vi "ExTestAdvDisp.vi"() -> ()   [LabVIEW 2010]
panel:
  out "After Pin zoom y":dbl format="%.2f"
  out "After Pin zoom x":dbl format="%.2f"
  out "zoom y":dbl format="%.2f"
  out "Zoom x":dbl format="%.2f"
  out "Cursor Y":u32
  out "Cursor X":u32
  in  "Full File Name":path
  out "error out":errorcluster
  in  "error in (no error)":errorcluster
  in  "SITKFULLDISPLAYLib.SITKFullDisplay":refnum<k7>(container)
  # "Browse match pattern is set to *.tif.  Modify this if different file type is needed."
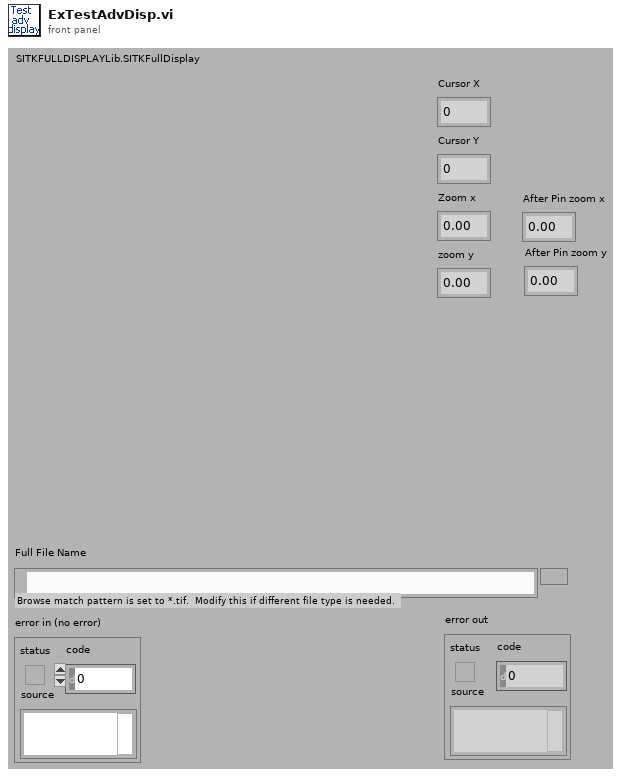
[diagram p1: front panel]
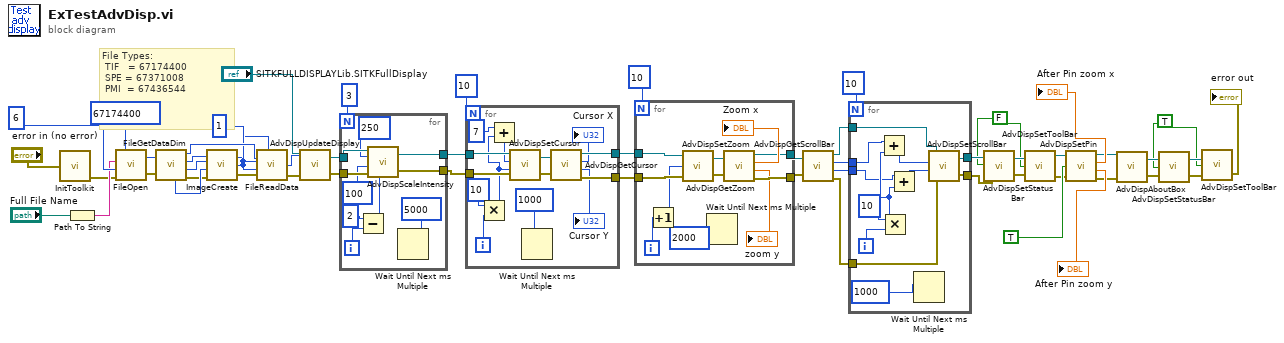
[diagram p0: block diagram]
diagram:
  w2 = TRUE
  w3 = FALSE
  w42 = 1
  # "File Types:\n TIF   = 67174400\n SPE = 67371008\n PMI  = 67436544"
  n1 = call <userlib>:"InitToolkit.vi"("error in"="error in (no error)") -> ("error out"=w38:errorcluster)
  n2 = Path To String(path="Full File Name") -> (string=w50:string)
  n3 = call <userlib>:"FileOpen.vi"("error in"=w38, "File Operations"=6, "FileName"=w50, "File Type"=67174400) -> ("error out"=w49:errorcluster, "File Handle"=w48:u32)
  n4 = call <userlib>:"FileGetDataDim.vi"("File Handle"=w48, "error in"=w49) -> ("Data Type"=w45:u32, "File Handle"=w43:u32, "X dim"=w47:u32, "Y dim"=w46:u32, "error out"=w44:errorcluster)  [unwired: 1 out]
  n5 = call <userlib>:"ImageCreate.vi"("X dimension"=w47, "Y dimension"=w46, "Data Type"=w45, "error in"=w44, "Number Of Frames"=w42) -> ("Image Handle"=w40:u32, "error out"=w41:errorcluster)
  n6 = call <userlib>:"FileReadData.vi"("File Handle"=w43, "Start Frame"=w42, "End Frame"=w42, "error in"=w41, "Image Handle"=w40) -> ("Image Handle"=w36:u32, "error out"=w35:errorcluster)  [unwired: 1 out]
  n7 = call <userlib>:"AdvDispUpdateDisplay.vi"("error in (no error)"=w35, "Image Handle"=w36, "SITKFULLDISPLAYLib.SITKFullDisplay"="SITKFULLDISPLAYLib.SITKFullDisplay") -> ("error out"=w34:errorcluster, "SITKFULLDISPLAYLib.SITKFullDisplay"=w33:refnum<k7>)  [unwired: 1 in]
  n8 = for {
    N: 3 -> [_]
    tunnel: [w63] -> w30
    tunnel: w34 -> [w62]
    tunnel: w33 -> [w61]
    tunnel: [w57] -> w29
    i -> [w54]
    n9 = Subtract(x=2, y=w54) -> (x-y=w56:i32)
    n10 = call <userlib>:"AdvDispScaleIntensity.vi"("SITKFULLDISPLAYLib.SITKFullDisplay"=w61, "High Intensity"=250, "Low Intensity"=100, "error in (no error)"=w62, "Type of Scale"=w56) -> ("SITKFULLDISPLAYLib.SITKFullDisplay"=w57:refnum<k7>, "error out"=w63:errorcluster)
    n11 = Wait Until Next ms Multiple(millisecond multiple=5000) -> ()  [unwired: 1 out]
  }
  n12 = for {
    N: 10 -> [_]
    tunnel: w30 -> [w74]
    tunnel: w29 -> [w77]
    tunnel: [w73] -> w27
    tunnel: [w72] -> w28
    i -> [w71]
    n13 = Multiply(x=10, y=w71) -> (x*y=w65:i32)
    n14 = Add(x=7, y=w65) -> (x+y=w64:i32)
    n15 = call <userlib>:"AdvDispSetCursor.vi"("error in (no error)"=w74, "Cursor Y"=w65, "Cursor X"=w64, "SITKFULLDISPLAYLib.SITKFullDisplay"=w77) -> ("error out"=w75:errorcluster, "SITKFULLDISPLAYLib.SITKFullDisplay"=w76:refnum<k7>)
    n16 = Wait Until Next ms Multiple(millisecond multiple=1000) -> ()  [unwired: 1 out]
    n17 = call <userlib>:"AdvDispGetCursor.vi"("SITKFULLDISPLAYLib.SITKFullDisplay"=w76, "error in (no error)"=w75) -> ("SITKFULLDISPLAYLib.SITKFullDisplay"=w72:refnum<k7>, "CursorX"=→"Cursor X":u32, "CursorY"=→"Cursor Y":u32, "error out"=w73:errorcluster)
  }
  n18 = for {
    N: 10 -> [_]
    tunnel: w28 -> [w84]
    tunnel: w27 -> [w83]
    tunnel: [w82] -> w24
    tunnel: [w78] -> w23
    i -> [w88]
    n19 = Increment(x=w88) -> (x+1=w80:i32)
    n20 = call <userlib>:"AdvDispSetZoom.vi"("error in (no error)"=w83, "Zoom Factor"=w80, "SITKFULLDISPLAYLib.SITKFullDisplay"=w84) -> ("error out"=w87:errorcluster, "SITKFULLDISPLAYLib.SITKFullDisplay"=w86:refnum<k7>)
    n21 = Wait Until Next ms Multiple(millisecond multiple=2000) -> ()  [unwired: 1 out]
    n22 = call <userlib>:"AdvDispGetZoom.vi"("SITKFULLDISPLAYLib.SITKFullDisplay"=w86, "error in (no error)"=w87) -> ("SITKFULLDISPLAYLib.SITKFullDisplay"=w78:refnum<k7>, "Zoom X"=→"Zoom x":dbl, "Zoom Y"=→"zoom y":dbl, "error out"=w82:errorcluster)
  }
  n23 = call <userlib>:"AdvDispGetScrollBar.vi"("SITKFULLDISPLAYLib.SITKFullDisplay"=w23, "error in (no error)"=w24) -> ("SITKFULLDISPLAYLib.SITKFullDisplay"=w19:refnum<k7>, "Scroll X position"=w21:i32, "Scroll Y position"=w22:i32, "error out"=w20:errorcluster)
  n24 = for {
    N: 10 -> [_]
    tunnel: w22 -> [w97]
    tunnel: w21 -> [w96]
    tunnel: w20 -> [w92]
    tunnel: w19 -> [w93]
    tunnel: [w91] -> w17
    tunnel: [w90] -> w16
    i -> [w100]
    n25 = Multiply(x=10, y=w100) -> (x*y=w98:i32)
    n26 = Add(x=w96, y=w98) -> (x+y=w94:i32)
    n27 = Add(x=w97, y=w98) -> (x+y=w95:i32)
    n28 = Wait Until Next ms Multiple(millisecond multiple=1000) -> ()  [unwired: 1 out]
    n29 = call <userlib>:"AdvDispSetScrollBar.vi"("error in (no error)"=w92, "Bar Y position"=w95, "Bar X position"=w94, "SITKFULLDISPLAYLib.SITKFullDisplay"=w93) -> ("error out"=w91:errorcluster, "SITKFULLDISPLAYLib.SITKFullDisplay"=w90:refnum<k7>)
  }
  n30 = call <userlib>:"AdvDispSetStatusBar.vi"("error in (no error)"=w17, "Status bar enable/disable"=w3, "SITKFULLDISPLAYLib.SITKFullDisplay"=w16) -> ("error out"=w15:errorcluster, "SITKFULLDISPLAYLib.SITKFullDisplay"=w14:refnum<k7>)
  n31 = call <userlib>:"AdvDispSetToolBar.vi"("error in (no error)"=w15, "Toolbar enable/disable"=w3, "SITKFULLDISPLAYLib.SITKFullDisplay"=w14) -> ("error out"=w13:errorcluster, "SITKFULLDISPLAYLib.SITKFullDisplay"=w12:refnum<k7>)
  n32 = call <userlib>:"AdvDispSetPin.vi"("SITKFULLDISPLAYLib.SITKFullDisplay"=w12, "Pin Enable"=TRUE, "error in (no error)"=w13) -> ("SITKFULLDISPLAYLib.SITKFullDisplay"=w8:refnum<k7>, "Zoom X"=→"After Pin zoom x":dbl, "Zoom Y"=→"After Pin zoom y":dbl, "error out"=w9:errorcluster)
  n33 = call <userlib>:"AdvDispAboutBox.vi"("error in (no error)"=w9, "SITKFULLDISPLAYLib.SITKFullDisplay"=w8) -> ("error out"=w7:errorcluster, "SITKFULLDISPLAYLib.SITKFullDisplay"=w6:refnum<k7>)
  n34 = call <userlib>:"AdvDispSetStatusBar.vi"("error in (no error)"=w7, "Status bar enable/disable"=w2, "SITKFULLDISPLAYLib.SITKFullDisplay"=w6) -> ("error out"=w5:errorcluster, "SITKFULLDISPLAYLib.SITKFullDisplay"=w4:refnum<k7>)
  n35 = call <userlib>:"AdvDispSetToolBar.vi"("error in (no error)"=w5, "Toolbar enable/disable"=w2, "SITKFULLDISPLAYLib.SITKFullDisplay"=w4) -> ("error out"=→"error out":errorcluster)  [unwired: 1 out]
